vi "Read Browse Button Rect.vi"(9 "Path in":refnum<class "Path.lvclass">) -> (3 "Path out":refnum<class "Path.lvclass">, 4 "Browse Button Rect":T1)   [LabVIEW 2014, in "Raspberry Pi Compatible Compiler for LabVIEW.lvlib" / "Path.lvclass"]
uses:
  Path.lvclass
  <vilib>/Utility/miscctls.llb/LVRectTypeDef.ctl
  Path.lvclass/Path.ctl
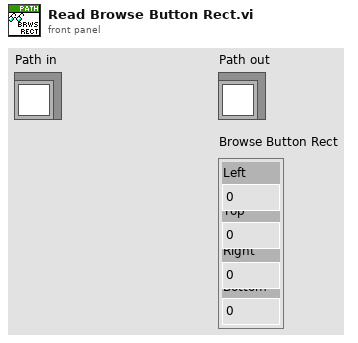
[diagram p1: front panel]
types:
  T1 = typedef "LVRectTypeDef.ctl" = cluster{"Left":i16, "Top":i16, "Right":i16, "Bottom":i16}
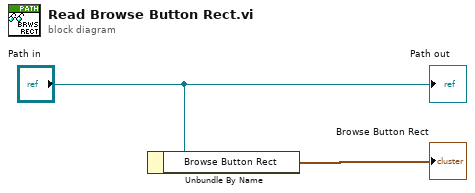
[diagram p0: block diagram]
diagram:
  n1 = Unbundle By Name("Path in") -> ("Browse Button Rect"=→"Browse Button Rect":T1)
  "Path out" <- "Path in"
